vi "OpenDevice.vi"(8 "错误输入（无错误）":errorcluster, 11 "DeviceType":T1=3 items=["PCI-CAN200"=7, "USB-CAN"=2, "USB-CAN200"=3]) -> (0 "错误输出":errorcluster, 2 "Result":bool, 3 "DeviceTypeOut":u16(ring)=7 items=["PCI-CAN200"=7])   [LabVIEW 2013]
uses:
  DevType.ctl
  VCI_CAN.dll
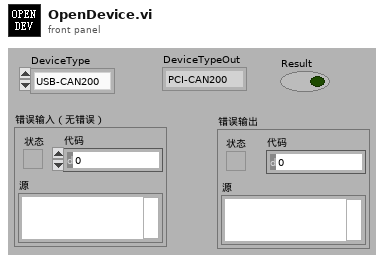
[diagram p1: front panel]
types:
  T1 = typedef "DevType.ctl" = u16
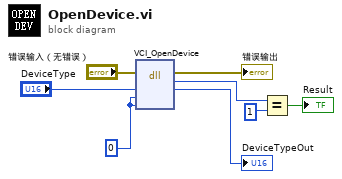
[diagram p0: block diagram]
diagram:
  w3 = 0
  n1 = dll-call lib="PTH1uabs D赛格T-BOXT-BOX TestSystem\nSourceCode五菱T-BOX TestSystemInstrumentDriversUSB-CANVCI_CAN.dll" fn="VCI_OpenDevice"(error in="错误输入（无错误）", "DevType"="DeviceType", "DevIndex"=w3, "Reserved"=w3) -> (error out=→"错误输出":errorcluster, "返回类型"=w4:u32, "DevType"=→"DeviceTypeOut":u32)  [unwired: 4 in, 1 out]
  n2 = Equal?(x=w4, y=u32 1) -> (x = y?=→"Result":bool)
